vi "5.PID-RT - DataLog - LED.vi"() -> ()   [LabVIEW 2014]
doc: "This example demonstrates how to simulate a general PID controller with alarms."
uses:
  vi.lib/Q-WaveSystems/QwaveSys Raspberry Pi for LabVIEW Home-Education/STM/_SubVIs/stm_MetaDataElement.ctl
  vi.lib/Q-WaveSystems/QwaveSys Raspberry Pi for LabVIEW Home-Education/CVT/_SubVIs/TypeDefs/cvt_Tag Configuration.ctl
  vi.lib/Q-WaveSystems/QwaveSys Raspberry Pi for LabVIEW Home-Education/CVT/_SubVIs/TypeDefs/cvt_Data Types.ctl
  <vilib>/Platform/TimedLoop/XDataNode/timing_clust.ctl
  <vilib>/Platform/TimedLoop/XDataNode/nitl_modes.ctl
  <vilib>/Platform/TimedLoop/XDataNode/wakeup.ctl
  <vilib>/MakerHub/LINX/Public/Peripherals/Digital/Digital Write N Chans.vi
  <vilib>/MakerHub/LINX/Private/Local IO/LinxDigitalWrite.vi
  <vilib>/MakerHub/LINX/Public/Utilities/Check Channel.vi
  vi.lib/Q-WaveSystems/QwaveSys Raspberry Pi for LabVIEW Home-Education/STM/TCP/STM Write Meta Data (TCP Ref).vi
  <vilib>/Utility/file.llb/Write To Spreadsheet File (DBL).vi
  vi.lib/Q-WaveSystems/QwaveSys Raspberry Pi for LabVIEW Home-Education/STM/TCP/STM Write Message (TCP).vi
  vi.lib/Q-WaveSystems/QwaveSys Raspberry Pi for LabVIEW Home-Education/STM/TCP/STM Get Connection Reference (TCP).vi
  <vilib>/MakerHub/LINX/Public/Utilities/Open Local.vi
  <vilib>/addons/control/pid/pid.llb/PID (DBL).vi
  <vilib>/MakerHub/LINX/Private/Utilties/Generate Error.vi
  <vilib>/platform/TimedLoop/XDataNode/XDataNode.xnode
  <vilib>/addons/control/pid/NI_PID_pid.lvlib
  <vilib>/Platform/TimedLoop/XDataNode/XDNodeRunTimeDep.lvlib
  vi.lib/Q-WaveSystems/QwaveSys Raspberry Pi for LabVIEW Home-Education/QwaveSys Raspberry Pi Library.lvlib
  <vilib>/MakerHub/LINX/LMH-LINX.lvlib
panel:
  in  "stop":bool
  in  "MIN":dbl(slide) scale=0.0..100.0
  in  "MAX":dbl(slide) scale=0.0..100.0
  out "Output (MV)":dbl(graph)
  out "Low Limit":bool
  out "High Limit":bool
  in  "SP:":dbl(slide)=54.966887417218544 min=0.0 max=0.0 scale=0.0..100.0
  out "MV:":dbl(slide)=100.0 scale=-100.0..100.0
  out "PV:":dbl(slide)=33.01408837398299 scale=0.0..100.0
  in  "PID gains":T1={"proportional gain (Kc)"=20.0, "integral time (Ti, min)"=0.008, "derivative time (Td, min)"=0.001} {"derivative time (Td, min)" format="%.3f"; "integral time (Ti, min)" format="%.3f"; "proportional gain (Kc)" format="%.3f"}
  out "Monitor Chart":cluster{"initial PV":dbl, "SP:":dbl, dbl, dbl}(graph)
  # "Overview: This example demonstrates how to simulate a general PID controller with alarms.\nInstructions:\n1. Run the VI and observe the Process Variable (PV) following the Setpoint (SP) value.\n2. Move the setpoint above or below the High Limit (HL) or Low Limit (LL). Verify the controls flashing when limits are reached.\n3. Change the Alarm limits to a value above or below if you are changing HL or LL, respectively and verify that the controller stop flashing.\n3. Click Stop to stop the VI."
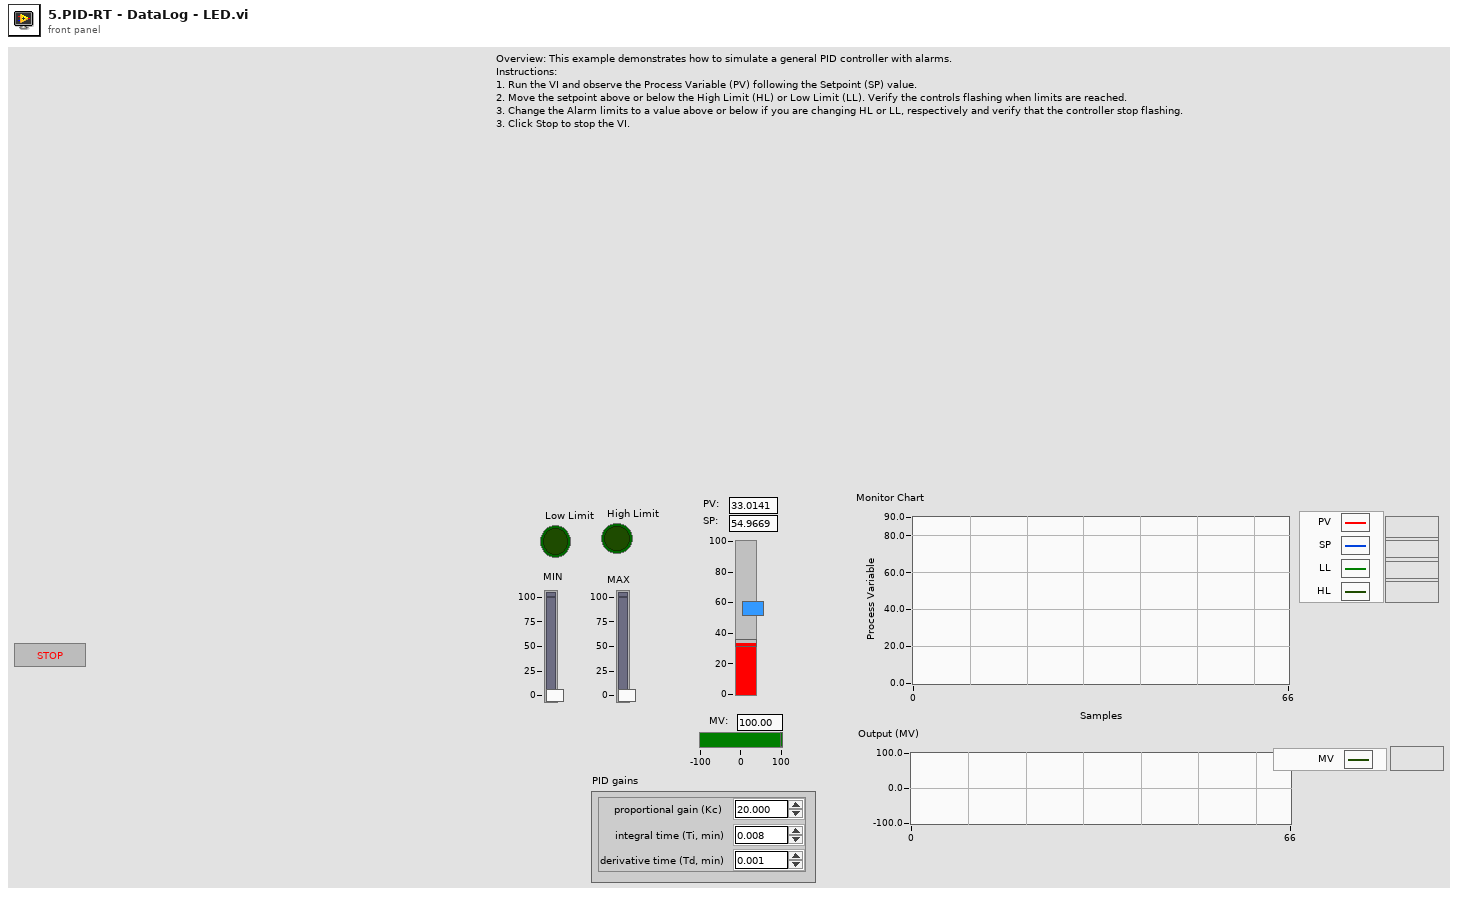
[diagram p1: front panel]
types:
  T1 = cluster{"proportional gain (Kc)":dbl, "integral time (Ti, min)":dbl, "derivative time (Td, min)":dbl}
  T2 = typedef "QwaveSys Raspberry Pi Library.lvlib/cvt_Tag Configuration.ctl" = cluster{"Name":string, "Data Type":T3, "Array":bool, "Size":u32, "Default":string, "Enum":string[], "Description":string}
  T3 = typedef "QwaveSys Raspberry Pi Library.lvlib/cvt_Data Types.ctl" = enum16{"Bool", "U8", "I32", "Double", "String", "Enum"}
  T4 = typedef "QwaveSys Raspberry Pi Library.lvlib/stm_MetaDataElement.ctl" = string
  T5 = typedef "LMH-LINX.lvlib/LINX Ref.ctl" = cluster{"IO":T6, "Interface":T7, "LINX Device Config":T8}
  T6 = typedef "LMH-LINX.lvlib/Platform.ctl" = enum16{"Remote", "Local"}
  T7 = typedef "LMH-LINX.lvlib/Interface.ctl" = enum16{"Serial", "TCP"}
  T8 = typedef "LMH-LINX.lvlib/Device.lvlib/LINX Device Config.ctl" = cluster{"Interface":T7, "COM Port":refnum<visa-resource-name>, "TCP Configuration":T9, "Device Family":u8, "Device ID":u8, "Device Name":string, "TCP Ref":refnum<k5>, "Channels":T10}
  T9 = typedef "LMH-LINX.lvlib/Device.lvlib/TCP Config.ctl" = cluster{"IP Address":string, "Port":u16}
  T10 = typedef "LMH-LINX.lvlib/Channels.ctl" = cluster{"DI":u8[], "DO":u8[], "AI":u8[], "AO":u8[], "PWM":u8[], "QE":u8[], "UART":u8[], "I2C 2":u8[], "SPI":u8[], "CAN":u8[], "Servo":u8[], "AI Ref (V)":dbl, "AI Resolution (Bits)":u8, "AO Ref (V)":dbl, "AO Resolution (Bits)":u8}
  T11 = typedef "XDNodeRunTimeDep.lvlib/timing_clust.ctl" = cluster{"Expected End [f-1]":u64, "Actual End [f-1]":u64, "Finished Late? [f-1]":bool, "Expected End [i-1]":u64, "Actual End [i-1]":u64, "Finished Late? [i-1]":bool, "Expected Start [i]":u64, "Actual Start [i]":u64, "Expected Start [f]":u64, "Actual Start [f]":u64, "Source Name":string, "Structure Name":string, "Period":i64, "Deadline":i64, "Offset":i64, "Start":i64, "Priority":i32, "Timeout":i32, "Mode":T12, "Wakeup Reason":T13, "Error":errorcluster, "Source Type":string, "Secondary Source Type":string, "Global End Time":u64, "Global Start Time":u64, "Frame Duration":u64, "Iteration Duration":u64, "Assigned CPU":i32, "I/O Scan Engine Mode":u32}
  T12 = typedef "XDNodeRunTimeDep.lvlib/nitl_modes.ctl" = enum32{"No Change", "Process missed periods, maintain original phase", "Discard missed periods, maintain original phase", "Process missed periods, ignore original phase", "Discard missed periods, ignore original phase"}
  T13 = typedef "XDNodeRunTimeDep.lvlib/wakeup.ctl" = enum32{"Normal", "Aborted", "Asynchronous wakeup", "Timing source error", "Timed loop error", "Timeout"}
  T14 = typedef "QwaveSys Raspberry Pi Library.lvlib/stm_TCP Connection Info.ctl" = cluster{"connection ID":refnum<k5>, "Meta data":T4[]}
  T15 = cluster{"static gain":dbl, "lag (min)":dbl, "dead cycles":dbl, "load %":dbl, "deadband":dbl, "noise level %":dbl, "initial PV":dbl, "initial PV 2":dbl}
  T16 = cluster{"Plant Output":dbl, "SP:":dbl, "MIN":dbl, "MAX":dbl}
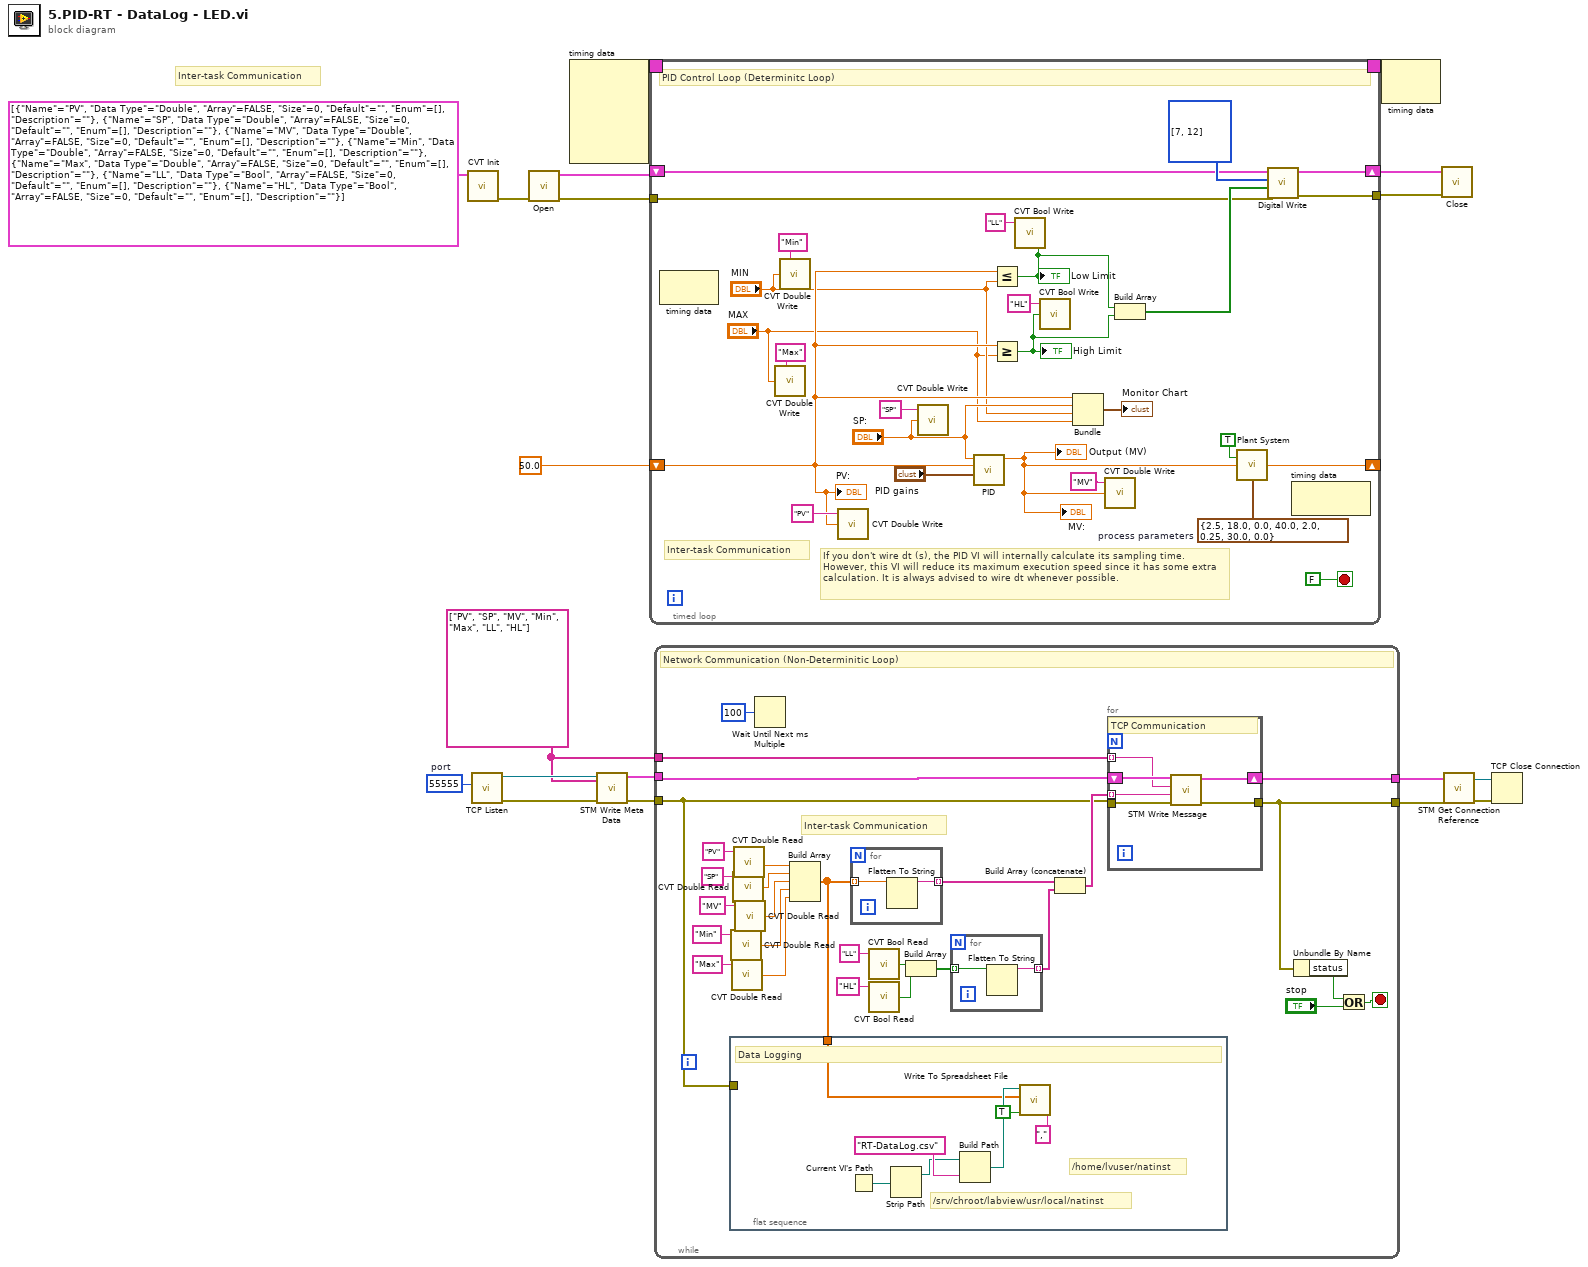
[diagram p0: block diagram]
diagram:
  w6 = T4[] ["PV", "SP", "MV", "Min", "Max", "LL", "HL"] ("Meta data")
  w16 = u16 55555  # port
  # "Inter-task Communication"
  n1 = call "CVT Init.vi"("Tag List"=T2[] [{"Name"="PV", "Data Type"=enum."Double", "Array"=FALSE, "Size"=0, "Default"="", "Enum"=[], "Description"=""}, {"Name"="SP", "Data Type"=enum."Double", "Array"=FALSE, "Size"=0, "Default"="", "Enum"=[], "Description"=""}, {"Name"="MV", "Data Type"=enum."Double", "Array"=FALSE, "Size"=0, "Default"="", "Enum"=[], "Description"=""}, {"Name"="Min", "Data Type"=enum."Double", "Array"=FALSE, "Size"=0, "Default"="", "Enum"=[], "Description"=""}, {"Name"="Max", "Data Type"=enum."Double", "Array"=FALSE, "Size"=0, "Default"="", "Enum"=[], "Description"=""}, {"Name"="LL", "Data Type"=enum."Bool", "Array"=FALSE, "Size"=0, "Default"="", "Enum"=[], "Description"=""}, {"Name"="HL", "Data Type"=enum."Bool", "Array"=FALSE, "Size"=0, "Default"="", "Enum"=[], "Description"=""}]) -> ("error out"=w1:errorcluster)  [unwired: 1 in, 9 out]
  n2 = call <vilib>:"TCP Listen.vi"("port"=w16) -> ("error out"=w14:errorcluster, "connection ID"=w15:refnum<k5>)  [unwired: 3 in, 6 out]
  n3 = call-poly <vilib>:"Open.vi"("Error In"=w1) -> ("Error Out"=w5:errorcluster, "LINX Resource"=w4:T5)  [unwired: 8 in, 1 out]
  n4 = node-c288() -> (w18:T11)  [unwired: 5 in]
  n5 = call-poly "STM Write Meta Data.vi"("Meta data"=w6, "error in"=w14, "connection ID"=w15) -> ("error out"=w12:errorcluster, "Connection Info Out"=w13:T14)  [unwired: 1 in, 6 out]
  n6 = timed-loop {
    shift-left: 50.0 ("Plant Output") -> [w38]
    shift-right: [w44] -> _
    timing: w18 -> [_]
    timing-out: [_] -> w17
    tunnel: w5 -> [w23]
    tunnel: [w20] -> w2
    shift-right: [w21] -> w3
    shift-left: w4 -> [w22]
    stop <- FALSE stop-if-true
    w42 = T15 {"static gain"=2.5, "lag (min)"=18.0, "dead cycles"=0.0, "load %"=40.0, "deadband"=2.0, "noise level %"=0.25, "initial PV"=30.0, "initial PV 2"=0.0}  # process parameters
    # "Inter-task Communication"
    # "If you don't wire dt (s), the PID VI will internally calculate its sampling time. However, this VI will reduce its maximum execution speed since it has some extra calculation. It is always advised to wire dt whenever possible."
    # "PID Control Loop (Determinitc Loop)"
    n7 = node-c288() -> ()  [unwired: 1 in, 1 out]
    n8 = call "CVT Double Write.vi"("Value"="MAX", "Tag Name"="Max") -> ()  [unwired: 3 in, 1 out]
    n9 = call "CVT Double Write.vi"("Value"="MIN", "Tag Name"="Min") -> ()  [unwired: 3 in, 1 out]
    n10 = call "CVT Double Write.vi"("Value"=w38, "Tag Name"="PV") -> ()  [unwired: 3 in, 1 out]
    n11 = call "CVT Double Write.vi"("Value"="SP:", "Tag Name"="SP") -> ()  [unwired: 3 in, 1 out]
    n12 = call-poly <vilib>:"PID.vi"("PID gains"="PID gains", "process variable"=w38, "setpoint"="SP:") -> ("output"=w34:dbl)  [unwired: 7 in, 1 out]
    "MV:" <- w34
    "Output (MV)" <- w34
    n13 = Less Or Equal?(x=w38, y="MIN") -> (x <= y?=w27:bool)
    "Low Limit" <- w27
    n14 = Greater Or Equal?(x=w38, y="MAX") -> (x >= y?=w26:bool)
    "High Limit" <- w26
    n15 = call "CVT Bool Write.vi"("Value"=w27, "Tag Name"="LL") -> ()  [unwired: 3 in, 1 out]
    n16 = call "CVT Bool Write.vi"("Value"=w26, "Tag Name"="HL") -> ()  [unwired: 3 in, 1 out]
    n17 = Bundle("Plant Output"=w38, "SP:"="SP:", "MIN"="MIN", "MAX"="MAX") -> (→"Monitor Chart":T16)  [unwired: 1 in]
    n18 = call "CVT Double Write.vi"("Value"=w34, "Tag Name"="MV") -> ()  [unwired: 3 in, 1 out]
    n19 = Build Array(w27, w26) -> (w25:bool[])
    n20 = call "Plant System.vi"("Integrator ?"=TRUE, "Plant Input"=w34, "process parameters"=w42) -> ("Plant Output"=w44:dbl)  [unwired: 12 in]
    n21 = call-poly <vilib>:"Digital Write.vi"("Error In"=w23, "Values"=w25, "DO Channels"=i32[] [7, 12], "LINX Resource"=w22) -> ("Error Out"=w20:errorcluster, "LINX Resource"=w21:T5)  [unwired: 6 in]
    n22 = node-c288() -> ()  [unwired: 1 in, 1 out]
    "PV:" <- w38
  }
  n23 = while {
    tunnel: w13 -> [w56]
    tunnel: w12 -> [w49]
    tunnel: [w55] -> w8
    tunnel: [w51] -> w7
    tunnel: w6 -> [w54]
    stop <- w50 stop-if-true
    # "Inter-task Communication"
    # "Network Communication (Non-Determinitic Loop)"
    n24 = flat-sequence {
      tunnel: w49 -> [_]
      tunnel: w48 -> [w77]
      frame #0 {
        # "/home/lvuser/natinst"
        # "/srv/chroot/labview/usr/local/natinst"
        # "Data Logging"
        n25 = Current VI's Path() -> (path=w82:path)
        n26 = Strip Path(path=w82) -> (stripped path=w80:path)  [unwired: 1 out]
        n27 = Build Path(base path=w80, name or relative path="RT-DataLog.csv") -> (appended path=w78:path)
        n28 = call-poly <vilib>:"Write To Spreadsheet File.vi"("delimiter (\\t)"="," ("delimiter (\\t)"), "append to file? (new file:F)"=TRUE, "1D data"=w77, "file path (dialog if empty)"=w78) -> ()  [unwired: 4 in, 1 out]
      }
    }
    n29 = call "CVT Double Read.vi"("Tag Name"="Min") -> ("Value"=w66:dbl)  [unwired: 3 in, 1 out]
    n30 = call "CVT Double Read.vi"("Tag Name"="Max") -> ("Value"=w65:dbl)  [unwired: 3 in, 1 out]
    n31 = call "CVT Double Read.vi"("Tag Name"="SP") -> ("Value"=w68:dbl)  [unwired: 3 in, 1 out]
    n32 = call "CVT Double Read.vi"("Tag Name"="PV") -> ("Value"=w73:dbl)  [unwired: 3 in, 1 out]
    n33 = call "CVT Double Read.vi"("Tag Name"="MV") -> ("Value"=w67:dbl)  [unwired: 3 in, 1 out]
    n34 = Wait Until Next ms Multiple(millisecond multiple=u32 100) -> ()  [unwired: 1 out]
    n35 = Build Array(w73, w68, w67, w66, w65) -> (w48:dbl[])
    n36 = for {
      tunnel: w48 -> [w86] mode=indexing
      tunnel: [w85] -> w62 mode=indexing
      n37 = Flatten To String(anything=w86) -> (data string=w85:string)  [unwired: 1 in, 4 out]
    }
    n38 = call "CVT Bool Read.vi"("Tag Name"="LL") -> ("Value"=w60:bool)  [unwired: 3 in, 1 out]
    n39 = call "CVT Bool Read.vi"("Tag Name"="HL") -> ("Value"=w59:bool)  [unwired: 3 in, 1 out]
    n40 = Build Array(w60, w59) -> (w61:bool[])
    n41 = for {
      tunnel: w61 -> [w84] mode=indexing
      tunnel: [w83] -> w58 mode=indexing
      n42 = Flatten To String(anything=w84) -> (data string=w83:string)  [unwired: 1 in, 4 out]
    }
    n43 = Build Array (concatenate)(w62, w58) -> (w57:string[])
    n44 = for {
      tunnel: [w91] -> w51
      tunnel: w49 -> [w90]
      tunnel: w57 -> [w88] mode=indexing
      shift-right: [w92] -> w55
      shift-left: w56 -> [w89]
      tunnel: w54 -> [w87] mode=indexing
      # "TCP Communication"
      n45 = call-poly "STM Write Message.vi"("error in (no error)"=w90, "Data"=w88, "Name"=w87, "Connection Info"=w89) -> ("error out"=w91:errorcluster, "Connection Info Out"=w92:T14)  [unwired: 1 in, 5 out]
    }
    n46 = Unbundle By Name(w51) -> ("status"=w52:bool)
    n47 = Or(x=w52, y="stop") -> (x .or. y?=w50:bool)
  }
  n48 = node-c288(w17) -> ()  [unwired: 1 out]
  n49 = call <vilib>:"Close.vi"("Error In"=w2, "LINX Resource"=w3) -> ()  [unwired: 9 in, 1 out]
  n50 = call-poly "STM Get Connection Reference.vi"("error in"=w7, "Connection Info"=w8) -> ("error out"=w10:errorcluster, "connection ID out"=w11:refnum<k5>)  [unwired: 8 out]
  n51 = TCP Close Connection(connection ID=w11, error in (no error)=w10) -> ()  [unwired: 3 out]
